vi "RunTestMotors.vi"() -> ()   [LabVIEW 2012]
panel:
  out "DIO13":bool
  out "DIO14":bool
  in  "V10":dbl
  in  "V9":dbl
  in  "V13":dbl
  in  "V12":dbl
  in  "V11":dbl
  in  "V7":dbl
  in  "V6":dbl
  in  "V8":dbl
  in  "V2V4":dbl
  in  "V1V3":dbl
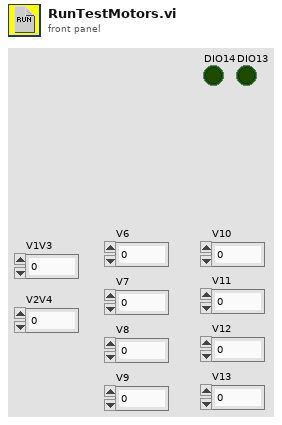
[diagram p1: front panel]
types:
  T1 = typedef "WPI_MotorControlDeviceRef.ctl" = cluster{"DeviceStatus":errorcluster, "Type":enum16{"PWM", "CAN"}, "PWM":cluster{"Digital Module":T2, "PWM Channel":T3, "DeadBand":T4}, "CAN":cluster{"Device Number":u8, "Control Mode":T5, "Semaphore":T6, "Max Vout":dbl}, "Invert":bool, "TransformRef":T7, "InvTransformRef":T7}
  T2 = typedef "FPGA_TypedefDigitalModule.ctl" = enum16{"Digital Module 1", "Digital Module 2"}
  T3 = typedef "FPGA_DIOPWMChannel.ctl" = enum8{"PWM 1", "PWM 2", "PWM 3", "PWM 4", "PWM 5", "PWM 6", "PWM 7", "PWM 8", "PWM 9", "PWM 10", "Invalid"}
  T4 = typedef "WPI_PWMDeadband.ctl" = cluster{"Name":string, "maxPositivePwm":i32, "minPositivePwm":i32, "centerPwm":i32, "maxNegativePwm":i32, "minNegativePwm":i32, "angularRange":u16}
  T5 = typedef "WPI_CANJaguar_ControlMode.ctl" = enum8{"Percent VBus", "Current", "Speed", "Position", "Voltage"}
  T6 = typedef "Semaphore RefNum" = refnum<k1>
  T7 = typedef "WPI_PWMTransform_ConPane.ctl" = refnum<vi>
  T8 = typedef "WPI_DigitalInputDevRef.ctl" = cluster{"DevStatus":errorcluster, "DIO Channel":T9, "Digital Module":T2}
  T9 = typedef "FPGA_DIOChannel.ctl" = enum8{"DIO 1", "DIO 2", "DIO 3", "DIO 4", "DIO 5", "DIO 6", "DIO 7", "DIO 8", "DIO 9", "DIO 10", "DIO 11", "DIO 12", "DIO 13", "DIO 14", "Invalid"}
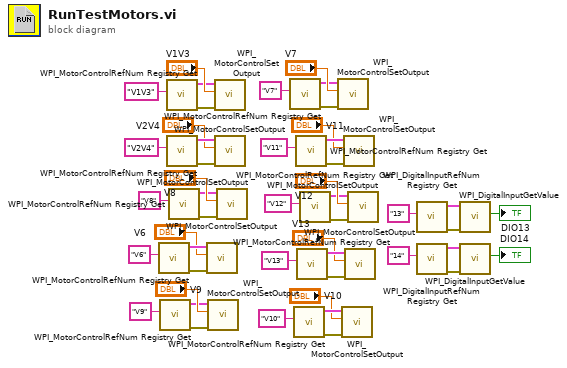
[diagram p0: block diagram]
diagram:
  n1 = call <vilib>:"WPI_MotorControlRefNum Registry Get.vi"("refnum name"="V6") -> ("error out"=w22:errorcluster, "MotorControlDevRef"=w23:T1)  [unwired: 9 in]
  n2 = call <vilib>:"WPI_MotorControlRefNum Registry Get.vi"("refnum name"="V9") -> ("error out"=w43:errorcluster, "MotorControlDevRef"=w42:T1)  [unwired: 9 in]
  n3 = call <vilib>:"WPI_MotorControlRefNum Registry Get.vi"("refnum name"="V1V3") -> ("error out"=w11:errorcluster, "MotorControlDevRef"=w10:T1)  [unwired: 9 in]
  n4 = call <vilib>:"WPI_MotorControlRefNum Registry Get.vi"("refnum name"="V2V4") -> ("error out"=w14:errorcluster, "MotorControlDevRef"=w15:T1)  [unwired: 9 in]
  n5 = call <vilib>:"WPI_MotorControlRefNum Registry Get.vi"("refnum name"="V8") -> ("error out"=w19:errorcluster, "MotorControlDevRef"=w18:T1)  [unwired: 9 in]
  n6 = call <vilib>:"WPI_MotorControlSetOutput.vi"("error in (no error)"=w22, "Output"="V6", "MotorControlDevRef"=w23) -> ()  [unwired: 6 in, 3 out]
  n7 = call <vilib>:"WPI_MotorControlSetOutput.vi"("error in (no error)"=w43, "Output"="V9", "MotorControlDevRef"=w42) -> ()  [unwired: 6 in, 3 out]
  n8 = call <vilib>:"WPI_MotorControlSetOutput.vi"("error in (no error)"=w11, "Output"="V1V3", "MotorControlDevRef"=w10) -> ()  [unwired: 6 in, 3 out]
  n9 = call <vilib>:"WPI_MotorControlSetOutput.vi"("error in (no error)"=w14, "Output"="V2V4", "MotorControlDevRef"=w15) -> ()  [unwired: 6 in, 3 out]
  n10 = call <vilib>:"WPI_MotorControlSetOutput.vi"("error in (no error)"=w19, "Output"="V8", "MotorControlDevRef"=w18) -> ()  [unwired: 6 in, 3 out]
  n11 = call <vilib>:"WPI_MotorControlRefNum Registry Get.vi"("refnum name"="V7") -> ("error out"=w27:errorcluster, "MotorControlDevRef"=w26:T1)  [unwired: 9 in]
  n12 = call <vilib>:"WPI_MotorControlRefNum Registry Get.vi"("refnum name"="V10") -> ("error out"=w46:errorcluster, "MotorControlDevRef"=w47:T1)  [unwired: 9 in]
  n13 = call <vilib>:"WPI_MotorControlRefNum Registry Get.vi"("refnum name"="V11") -> ("error out"=w30:errorcluster, "MotorControlDevRef"=w31:T1)  [unwired: 9 in]
  n14 = call <vilib>:"WPI_MotorControlRefNum Registry Get.vi"("refnum name"="V13") -> ("error out"=w38:errorcluster, "MotorControlDevRef"=w39:T1)  [unwired: 9 in]
  n15 = call <vilib>:"WPI_MotorControlRefNum Registry Get.vi"("refnum name"="V12") -> ("error out"=w35:errorcluster, "MotorControlDevRef"=w34:T1)  [unwired: 9 in]
  n16 = call <vilib>:"WPI_MotorControlSetOutput.vi"("error in (no error)"=w27, "Output"="V7", "MotorControlDevRef"=w26) -> ()  [unwired: 6 in, 3 out]
  n17 = call <vilib>:"WPI_MotorControlSetOutput.vi"("error in (no error)"=w46, "Output"="V10", "MotorControlDevRef"=w47) -> ()  [unwired: 6 in, 3 out]
  n18 = call <vilib>:"WPI_MotorControlSetOutput.vi"("error in (no error)"=w30, "Output"="V11", "MotorControlDevRef"=w31) -> ()  [unwired: 6 in, 3 out]
  n19 = call <vilib>:"WPI_MotorControlSetOutput.vi"("error in (no error)"=w38, "Output"="V13", "MotorControlDevRef"=w39) -> ()  [unwired: 6 in, 3 out]
  n20 = call <vilib>:"WPI_MotorControlSetOutput.vi"("error in (no error)"=w35, "Output"="V12", "MotorControlDevRef"=w34) -> ()  [unwired: 6 in, 3 out]
  n21 = call <vilib>:"WPI_DigitalInputRefNum Registry Get.vi"("refnum name"="13") -> ("error out"=w8:errorcluster, "DigitalInputDevRef"=w7:T8)  [unwired: 9 in]
  n22 = call <vilib>:"WPI_DigitalInputRefNum Registry Get.vi"("refnum name"="14") -> ("error out"=w3:errorcluster, "DigitalInputDevRef"=w4:T8)  [unwired: 9 in]
  n23 = call <vilib>:"WPI_DigitalInputGetValue.vi"("error in (no error)"=w8, "DigitalInputDevRef"=w7) -> ("Value"=→"DIO13":bool)  [unwired: 7 in, 2 out]
  n24 = call <vilib>:"WPI_DigitalInputGetValue.vi"("error in (no error)"=w3, "DigitalInputDevRef"=w4) -> ("Value"=→"DIO14":bool)  [unwired: 7 in, 2 out]
